vi "Open Center and Close FP.vi"(7 "Active？":bool=TRUE, 8 "错误输入（无错误）":errorcluster, 9 "State":T1(ring)=enum."Standard", 10 "Mode":enum16{"Open", "Close", "Center"}(ring), 11 "VI Ref In":refnum<vi>) -> (0 "错误输出":errorcluster, 3 "Ref Out":refnum<vi>)   [LabVIEW 2012, in "VIRef.lvlib"]
uses:
  VIRef.lvlib
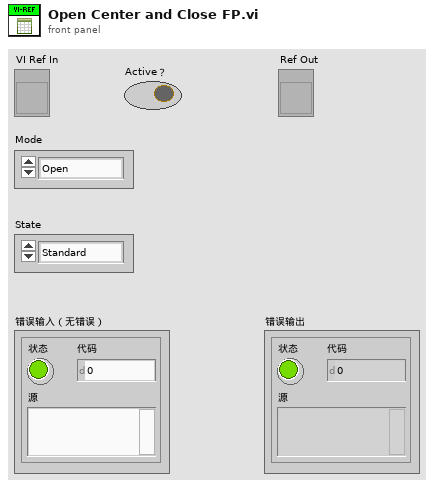
[diagram p1: front panel]
types:
  T1 = enum32{"Invalid", "Standard", "Closed", "Hidden", "Minimized", "Maximized"}
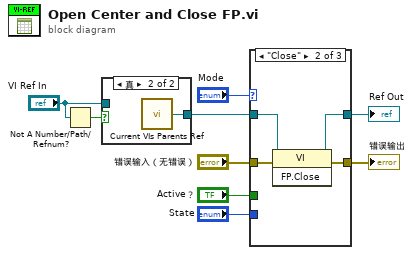
[diagram p0: block diagram]
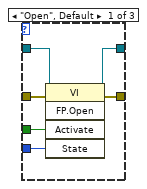
[diagram p2: hidden frame]
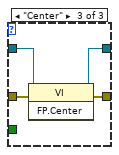
[diagram p3: hidden frame]
diagram:
  n1 = Not A Number/Path/Refnum?(number/path/refnum="VI Ref In") -> (NaN/Path/Refnum?=w8:bool)
  n2 = case shown="真" w8 {
    tunnel: [w10 w11] -> w4
    tunnel: "VI Ref In" -> [w10 _]
    frame False {
    }
    frame True {
      n3 = call "Current VIs Parents Ref.vi"() -> ("Calling VI's Reference"=w11:refnum<vi>)  [unwired: 2 in]
    }
  }
  n4 = case shown="\"Close\"" "Mode" {
    tunnel: "错误输入（无错误）" -> [w17 w21 w24]
    tunnel: [w16 w19 w23] -> w5
    tunnel: w4 -> [w15 w20 w25]
    tunnel: [w14 w18 w22] -> w3
    tunnel: "Active？" -> [w13 _ _]
    tunnel: "State" -> [w12 _ _]
    frame "Open", Default {
      n5 = invoke class="VI" method="FP.Open"(reference=w15, error in=w17, "Activate"=w13, "State"=w12) -> (reference out=w14:refnum<vi>, error out=w16:errorcluster)  [unwired: 1 in, 3 out]
    }
    frame "Close" {
      n6 = invoke class="VI" method="FP.Close"(reference=w20, error in=w21) -> (reference out=w18:refnum<vi>, error out=w19:errorcluster)  [unwired: 1 in, 1 out]
    }
    frame "Center" {
      n7 = invoke class="VI" method="FP.Center"(reference=w25, error in=w24) -> (reference out=w22:refnum<vi>, error out=w23:errorcluster)  [unwired: 1 in, 1 out]
    }
  }
  "错误输出" <- w5
  "Ref Out" <- w3
